vi "NotifyOwner(SelfTermination).vi"(8 "error in (no error)":errorcluster, 11 "SMO in":refnum<class "SMO.lvclass">) -> (0 "error out":errorcluster, 3 "SMO out":refnum<class "SMO.lvclass">)   [LabVIEW 2021, in "smo.lvlib" / "SMO.lvclass"]
uses:
  SMO.lvclass
  Support/Attribute.Owner/Attribute.Owner.lvclass
  SMO.lvclass/SMO.ctl
  ReftoDVR--SMO.vi
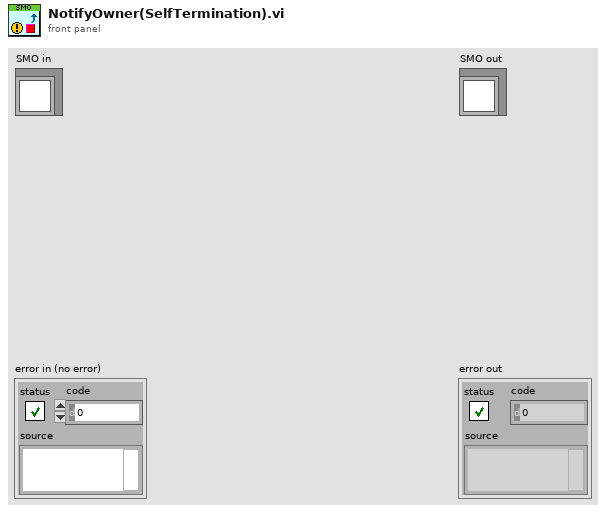
[diagram p1: front panel]
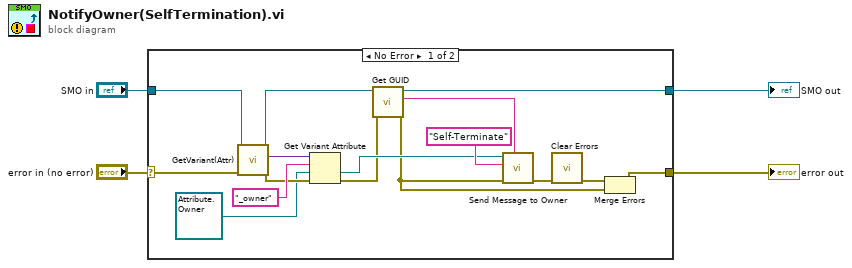
[diagram p0: block diagram]
diagram:
  n1 = case shown="No Error" "error in (no error)" {
    selector: "error in (no error)" -> [w11 w22]
    tunnel: [w19 w22] -> w3
    tunnel: [w18 w21] -> w1
    tunnel: "SMO in" -> [w10 w21]
    frame No Error {
      n2 = call "GetVariant(Attr).vi"("error in (no error)"=w11, "SMO in"=w10) -> ("error out"=w13:errorcluster, "[Attributes]"=w15:variant, "SMO out"=w9:refnum<class "SMO.lvclass">)  [unwired: 7 in]
      n3 = Get Variant Attribute(Variant=w15, name="_owner", default value (empty Variant)=refnum<class "Attribute.Owner.lvclass"> refnum ("Attribute.Owner.lvclass"), error in=w13) -> (value=w8:refnum<class "Attribute.Owner.lvclass">, error out=w7:errorcluster)  [unwired: 2 out]
      n4 = call "Get GUID.vi"("error in (no error)"=w7, "SMO"=w9) -> ("error out"=w5:errorcluster, "GUID"=w17:string, "SMO out"=w18:refnum<class "SMO.lvclass">)  [unwired: 7 in]
      n5 = call "Send Message to Owner.vi"("GUID"=w17, "error in (no error)"=w5, "Message"="Self-Terminate", "Attribute.Owner in"=w8) -> ("error out"=w20:errorcluster)  [unwired: 6 in, 1 out]
      n6 = call <vilib>:"Clear Errors.vi"("error in (no error)"=w20) -> ("error out"=w6:errorcluster)  [unwired: 5 in, 1 out]
      n7 = Merge Errors(w6, w5) -> (w19:errorcluster)
    }
    frame Error {
    }
  }
  "error out" <- w3
  "SMO out" <- w1
